vi "Fetch Loop.vi"(11 "niInstr Multirecord Acquisition Common v1 FPGA in":refnum<class "niInstr Multirecord Acquisition Common v1 FPGA.lvclass">) -> ()   [LabVIEW 2021]
uses:
  <instrlib>/_niInstr/Multirecord Acquisition/Common/v1/FPGA/niInstr Multirecord Acquisition Common v1 FPGA.lvclass
  C:/Program Files (x86)/National Instruments/LabVIEW 2021/instr.lib/_niInstr/Multirecord Acquisition/Interface/v1/FPGA/niInstr Multirecord Acquisition v1 FPGA.lvclass
  <vilib>/Platform/TimedLoop/XDataNode/timing_clust.ctl
  <vilib>/Platform/TimedLoop/XDataNode/nitl_modes.ctl
  <vilib>/Platform/TimedLoop/XDataNode/wakeup.ctl
  <vilib>/rvi/Emulation/niFpgaSctlEmulationGetInTimedLoop.vi
  <vilib>/rvi/Emulation/niFpgaEmulationReportErrorSimple.vi
  <vilib>/rvi/Emulation/niFpgaGetClockAttributes.vi
  <vilib>/rvi/Emulation/niFpgaCriticalErrorInLSC.vi
  <instrlib>/_niInstr/Multirecord Acquisition/Interface/v1/FPGA/Private/Retrieve Record U16 Wrapper.vi
  <instrlib>/_niInstr/Multirecord Acquisition/Interface/v1/FPGA/Private/Write to Fetch DMA FIFO U16 Wrapper.vi
  <vilib>/Platform/TimedLoop/XDataNode/XDataNode.xnode
  <vilib>/Platform/TimedLoop/XDataNode/XDNodeRunTimeDep.lvlib
  <instrlib>/_niInstr/Multirecord Acquisition/Interface/v1/FPGA/niInstr Multirecord Acquisition v1 FPGA.lvclass
  C:/Program Files (x86)/National Instruments/LabVIEW 2021/instr.lib/_niInstr/Multirecord Acquisition/Common/v1/FPGA/niInstr Multirecord Acquisition Common v1 FPGA.lvclass
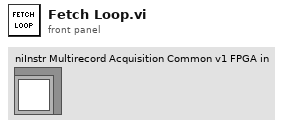
[diagram p1: front panel]
types:
  T1 = typedef "XDNodeRunTimeDep.lvlib/timing_clust.ctl" = cluster{"Expected End [f-1]":u64, "Actual End [f-1]":u64, "Finished Late? [f-1]":bool, "Expected End [i-1]":u64, "Actual End [i-1]":u64, "Finished Late? [i-1]":bool, "Expected Start [i]":u64, "Actual Start [i]":u64, "Expected Start [f]":u64, "Actual Start [f]":u64, "Source Name":string, "Structure Name":string, "Period":i64, "Deadline":i64, "Offset":i64, "Start":i64, "Priority":i32, "Timeout":i32, "Mode":T2, "Wakeup Reason":T3, "Error":errorcluster, "Source Type":string, "Secondary Source Type":string, "Global End Time":u64, "Global Start Time":u64, "Frame Duration":u64, "Iteration Duration":u64, "Assigned CPU":i32, "I/O Scan Engine Mode":u32}
  T2 = typedef "XDNodeRunTimeDep.lvlib/nitl_modes.ctl" = enum32{"No Change", "Process missed periods, maintain original phase", "Discard missed periods, maintain original phase", "Process missed periods, ignore original phase", "Discard missed periods, ignore original phase"}
  T3 = typedef "XDNodeRunTimeDep.lvlib/wakeup.ctl" = enum32{"Normal", "Aborted", "Asynchronous wakeup", "Timing source error", "Timed loop error", "Timeout"}
  T4 = typedef "niInstr Multirecord Acquisition v1 FPGA.lvclass/Retrieve Data Info.ctl" = cluster{"read request size (bits)":u64, "valid data offset (bits)":u16, "valid data size (bits)":u16, "first sample of request":bool, "last sample of request":bool, "Token":T5}
  T5 = typedef "niInstr Types v1 Shared.lvlib/Token.ctl" = cluster{"identifier":u8, "value":u32}
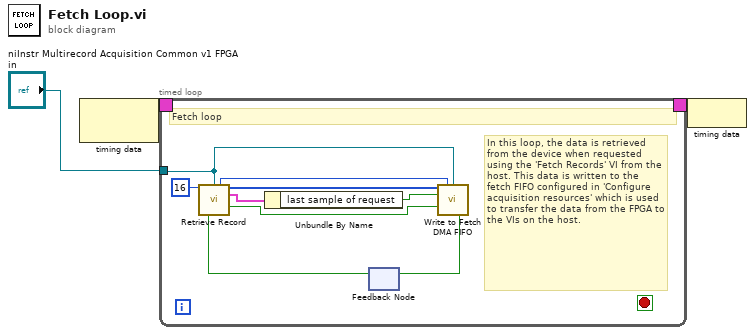
[diagram p0: block diagram]
diagram:
  n1 = node-c288() -> (w3:T1)  [unwired: 1 in]
  n2 = timed-loop {
    timing: w3 -> [_]
    timing-out: [_] -> w2
    tunnel: "niInstr Multirecord Acquisition Common v1 FPGA in" -> [w12]
    stop <- _ stop-if-true
    # "In this loop, the data is retrieved from the device when requested using the 'Fetch Records' VI from the host. This data is written to the fetch FIFO configured in 'Configure acquisition resources' which is used to transfer the data from the FPGA to the VIs on the host."
    # "Fetch loop"
    n3 = feedback #1() -> (w10:bool)  [unwired: 1 in]
    n4 = call-poly <instrlib>:"Retrieve Record.vi"("output array size"=u16 16, "acquisition resources"=w12, "ready for output"=w10) -> ("channels"=w5:u8, "data"=w8:u16[], "retrieve data info"=w7:T4, "output valid"=w9:bool)  [unwired: 9 in]
    n5 = Unbundle By Name(w7) -> ("last sample of request"=w6:bool)
    n6 = call-poly <instrlib>:"Write to Fetch DMA FIFO.vi"("data"=w8, "channels"=w5, "acquisition resources"=w12, "last sample of request"=w6, "input valid"=w9) -> ("ready for input"=w11:bool)  [unwired: 10 in]
    n7 = feedback-in #1(w11) -> ()
  }
  n8 = node-c288(w2) -> ()
